vi "Write State Update Rate.vi"(8 "error in (no error)":errorcluster, 10 "State Update Rate":dbl, 11 "RDS State Tracker in":refnum<class "RDS State Tracker.lvclass">) -> (0 "error out":errorcluster, 3 "RDS State Tracker out":refnum<class "RDS State Tracker.lvclass">)   [LabVIEW 2015, in "RDS State Tracker.lvlib" / "RDS State Tracker.lvclass"]
uses:
  RDS State Tracker.lvclass
  RDS State Tracker.lvclass/RDS State Tracker.ctl
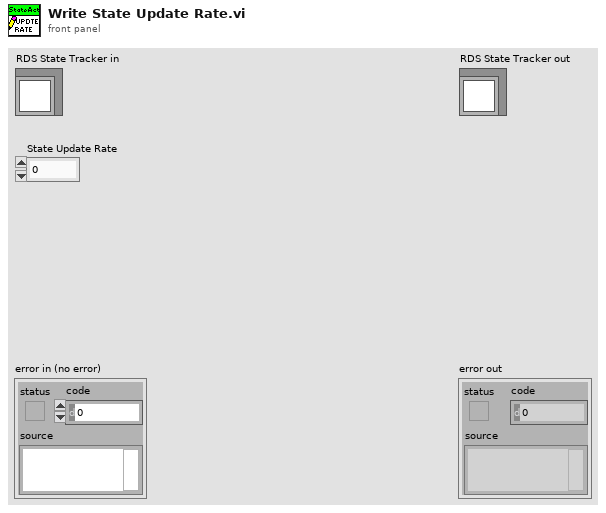
[diagram p1: front panel]
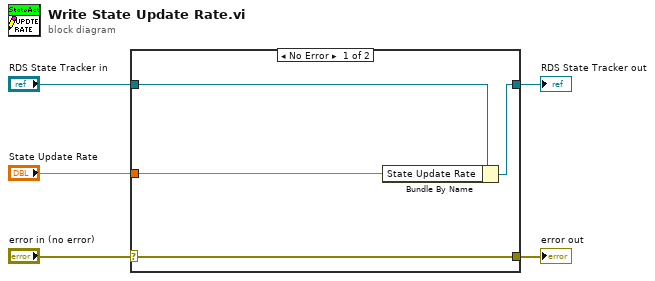
[diagram p0: block diagram]
diagram:
  n1 = case shown="No Error" "error in (no error)" {
    selector: "error in (no error)" -> [w9 w10]
    tunnel: [w9 w10] -> w4
    tunnel: [w7 w11] -> w2
    tunnel: "RDS State Tracker in" -> [w8 w11]
    tunnel: "State Update Rate" -> [w6 _]
    frame No Error {
      n2 = Bundle By Name(cluster=w8, "State Update Rate"=w6) -> (w7:refnum<class "RDS State Tracker.lvclass">)
    }
    frame Error {
    }
  }
  "error out" <- w4
  "RDS State Tracker out" <- w2
